vi "Solid Dilution Control-7.vi"() -> ()   [LabVIEW 2011]
uses:
  <vilib>/Instr/_visa.llb/VISA Configure Serial Port (Instr).vi
panel:
  out "(SCB) Raw":dbl
  out "Target = Soln Size?":bool=TRUE
  in  "Fill Target":dbl=450.0
  out "Hydration (g)":dbl
  in  "SIM MASS":dbl=900.0
  in  "real":bool=TRUE
  out "# of Rows Saved":i32
  in  "Tab Control":enum32{"DISPLAY", "CONFIGURE"}(tab)
  in  "Settings":T1={"ON Settings"={"Enable Dynamic Setpoint?"=TRUE, "Enable Dynamic Dispense Time?"=TRUE, "Enable Drain Rate Functions"=TRUE, "Dispense Sample Time (s)"=0.1, "Mass Average Samples"=20, "ON Timeout (sec)"=300.0, "1st Setpoint (% of Target)"=90.0, "2nd Setpoint (% of Target)"=95.0, "3rd Setpoint (% of Target)"=100.0, "Measure Dispense Delay (sec)"=10.0, "Minimum Spray Time (s)"=2.0, "Pump Reverse Time (s)"=10.0}, "OFF Settings"={"Drain Sample Time (s)"=0.1, "Drain Rate Ave Size"=100, "Drain Rate Limits (± g/sec)"=100.0, "Level Slope Range (± g/sec)"=0.05, "OFF Timeout (sec)"=300.0, "Near SP Slope Level (± g/sec)"=0.005, "Near Setpoint Threshold (%)"=99.0}, "Overshoot Settings"={"Time Limit (s)"=30.0, "Container MAX (g)"=1500.0, "Max FILL Slope (+/- g/sec)"=100.0, "% Overshot to Enable (>)"=3.0}, "FILL Timeout (s)"=300.0, "Full \nSettle Time (s)"=30.0, "Pre-Hydrate \nSpray Time (s)"=0.0, "Pre-Hydrate \nWait Time (s)"=10.0, "m Value "=1.0, "b Value"=0.0, "Enable Overshoot Adjust?"=FALSE} {"ON Settings"."Pump Reverse Time (s)" min=0.0 max=60.0; "OFF Settings"."Near SP Slope Level (± g/sec)" format="%.3g"; "OFF Settings"."Level Slope Range (± g/sec)" format="%.3g"}
  out "Values":T2 {"Drain Time (s)" format="%.2f"; "Drain Rate (g/sec)" format="%.2f"; "Spray Mass Loss (g)" format="%.2f"; "Time Elapsed (s)" format="%.2f"; "Time Target (s)" format="%.2f"; "Dynamic Setpoint (g)" format="%.2f"; "Static Setpoint (g)" format="%.2f"; "Grams to Setpoint" format="%.2f"; "Adjusted Mass (g)" format="%.2f"; "Dispense Rate (g/sec)" format="%.2f"; "Fill Mass (g)" format="%.2f"; "Fill Rate (g/sec)" format="%.2f"}
  in  "Settings Button":bool
  in  "START Dispense":bool
  in  "STOP Dispense":bool
  in  "Fill Setpoint (g)":dbl
  in  "Dispense Setpoint (%)":dbl=10.0
  out "Mass Chart":T3(graph)={"Grams (SCB)"=0.0, "Fill Target"=450.0, "Dispense Target"=0.0}
  out "Signals":T4={"Dispense"=FALSE, "Fill"=FALSE, "Spray"=FALSE, "Drain"=TRUE, "Complete"=FALSE, "Fill Error"=FALSE, "Disp. Error"=FALSE, "Fill Timeout"=FALSE, "Disp. Timeout"=FALSE, "Purge"=TRUE}
  in  "Solution Size (g)":dbl=500.0
  out "Dispense Mode":T5(ring)
  in  "Tare":bool
  out "Relay Status":T6
  in  "Save Interval (s)":dbl=1.0
  in  "Write/Read Wait (ms)":u32=100
  in  "Event Loop Wait (ms)":i32=5000
  in  "File Path Input":path
  out "SCB Error":errorcluster={"status"=TRUE, "code"=-1073807343, "source"="Property Node (arg 1) in Read SCB via ESP (SubVI).vi->Solid Dilution Control-7.vi"}
  out "SCB Output":T7
  in  "SCB COM Port":refnum<visa-resource-name>="COM5"
  in  "SCB Baud Rate":u32=9600
  out "SCB Com Error":errorcluster={"status"=TRUE, "code"=-1073807343, "source"="Property Node (arg 1) in VISA Configure Serial Port (Instr).vi->Solid Dilution Control-7.vi"}
  out "Save Error":errorcluster caption="Error Output"
  out "Weight (Grams)":dbl format="%.2f"
  out "Product Values":T8
  out "Spray Count":i32
  in  "9481 Name":tag="cDAQ3Mod1"
  out "9481 Error":errorcluster
  in  "Relay Control":T6
  out "Event Loop":i32=4
  out "Main Loop":i32=599
  out "Save Loop":i32=64
  out "DAQ/SCB Loop":i32=57
  in  "Save (Enable/Signal)":bool
  in  "STOP PROGRAM":bool
  # "SOLID DILUTION CONTROL SYSTEM"
  # "Program Last Updated 6-28-2012"
  # "SAVE\nENABLE"
  # "Blake Otting - Systems Engineering Lab - 2009"
  # "DISPENSE CONTROL"
  # "ONLY ADJUST\nBOLD VALUES!"
  # "Corrected Mass = SDC Mass * m + b"
  # "Ch0"
  # "Ch1"
  # "Ch2"
  # "Ch3"
  # "RELAY MODULE"
  # "Manual Control"
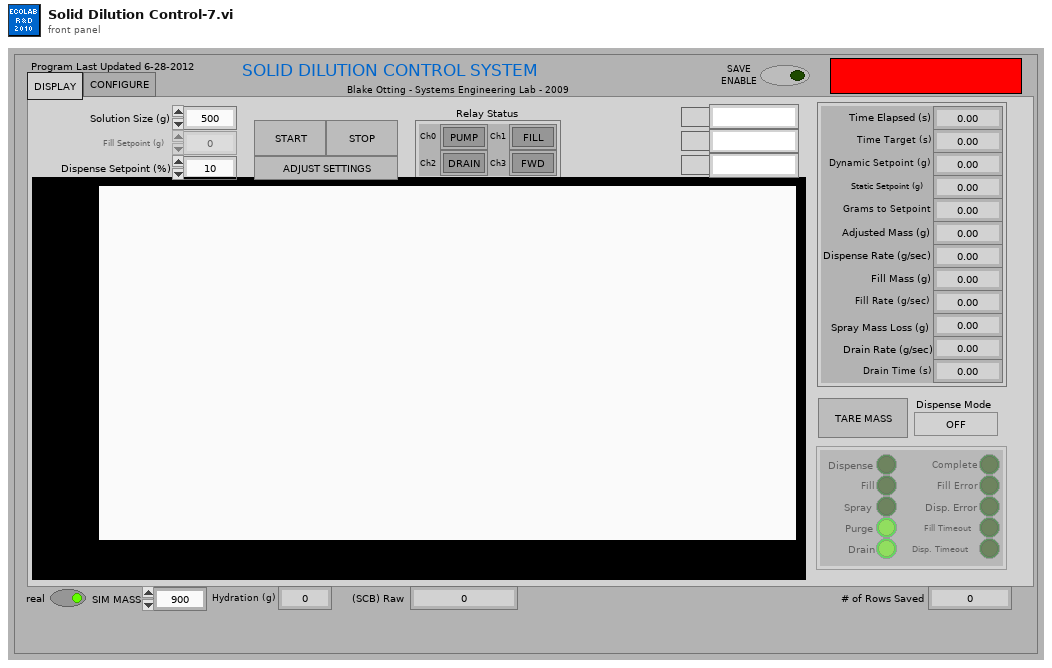
[diagram p1: front panel]
types:
  T1 = cluster{"ON Settings":cluster{"Enable Dynamic Setpoint?":bool, "Enable Dynamic Dispense Time?":bool, "Enable Drain Rate Functions":bool, "Dispense Sample Time (s)":dbl, "Mass Average Samples":i32, "ON Timeout (sec)":dbl, "1st Setpoint (% of Target)":dbl, "2nd Setpoint (% of Target)":dbl, "3rd Setpoint (% of Target)":dbl, "Measure Dispense Delay (sec)":dbl, "Minimum Spray Time (s)":dbl, "Pump Reverse Time (s)":dbl}, "OFF Settings":cluster{"Drain Sample Time (s)":dbl, "Drain Rate Ave Size":i32, "Drain Rate Limits (± g/sec)":dbl, "Level Slope Range (± g/sec)":dbl, "OFF Timeout (sec)":dbl, "Near SP Slope Level (± g/sec)":dbl, "Near Setpoint Threshold (%)":dbl}, "Overshoot Settings":cluster{"Time Limit (s)":dbl, "Container MAX (g)":dbl, "Max FILL Slope (+/- g/sec)":dbl, "% Overshot to Enable (>)":dbl}, "FILL Timeout (s)":dbl, "Full \nSettle Time (s)":dbl, "Pre-Hydrate \nSpray Time (s)":dbl, "Pre-Hydrate \nWait Time (s)":dbl, "m Value ":dbl, "b Value":dbl, "Enable Overshoot Adjust?":bool}
  T2 = cluster{"Time Elapsed (s)":dbl, "Time Target (s)":dbl, "Dynamic Setpoint (g)":dbl, "Static Setpoint (g)":dbl, "Grams to Setpoint":dbl, "Adjusted Mass (g)":dbl, "Dispense Rate (g/sec)":dbl, "Fill Mass (g)":dbl, "Fill Rate (g/sec)":dbl, "Spray Mass Loss (g)":dbl, "Drain Rate (g/sec)":dbl, "Drain Time (s)":dbl}
  T3 = cluster{"Grams (SCB)":dbl, "Fill Target":dbl, "Dispense Target":dbl}
  T4 = cluster{"Dispense":bool, "Fill":bool, "Spray":bool, "Drain":bool, "Complete":bool, "Fill Error":bool, "Disp. Error":bool, "Fill Timeout":bool, "Disp. Timeout":bool, "Purge":bool}
  T5 = enum16{"OFF", "INITIAL", "FILL", "DISPENSE", "ADJUST"}
  T6 = cluster{"PUMP ON":bool, "BASIN FILL":bool, "BASIN DRAIN":bool, "PUMP DIRECTION":bool}
  T7 = cluster{"Sequence #":string, "Weight":string, "Status":string, "CRC & EOT":string}
  T8 = cluster{"Drain Delta":dbl, "Spray Delta":dbl, "Dispense Delta":dbl}
  T9 = enum8{"Enabled", "Disabled", "Disabled and Grayed Out"}
  T10 = cluster{"Grams (SCB)":dbl, "Fill Target":dbl, "Dispense Target":dbl}[]
  T11 = cluster{"SPRAY":bool, "FILL":bool, "DRAIN":bool, "DIRECTION":bool}
  T12 = cluster{"Row Limit":i32, "Default File Name":string, "New File Daily?":bool, "Manual Save Interval?":bool}
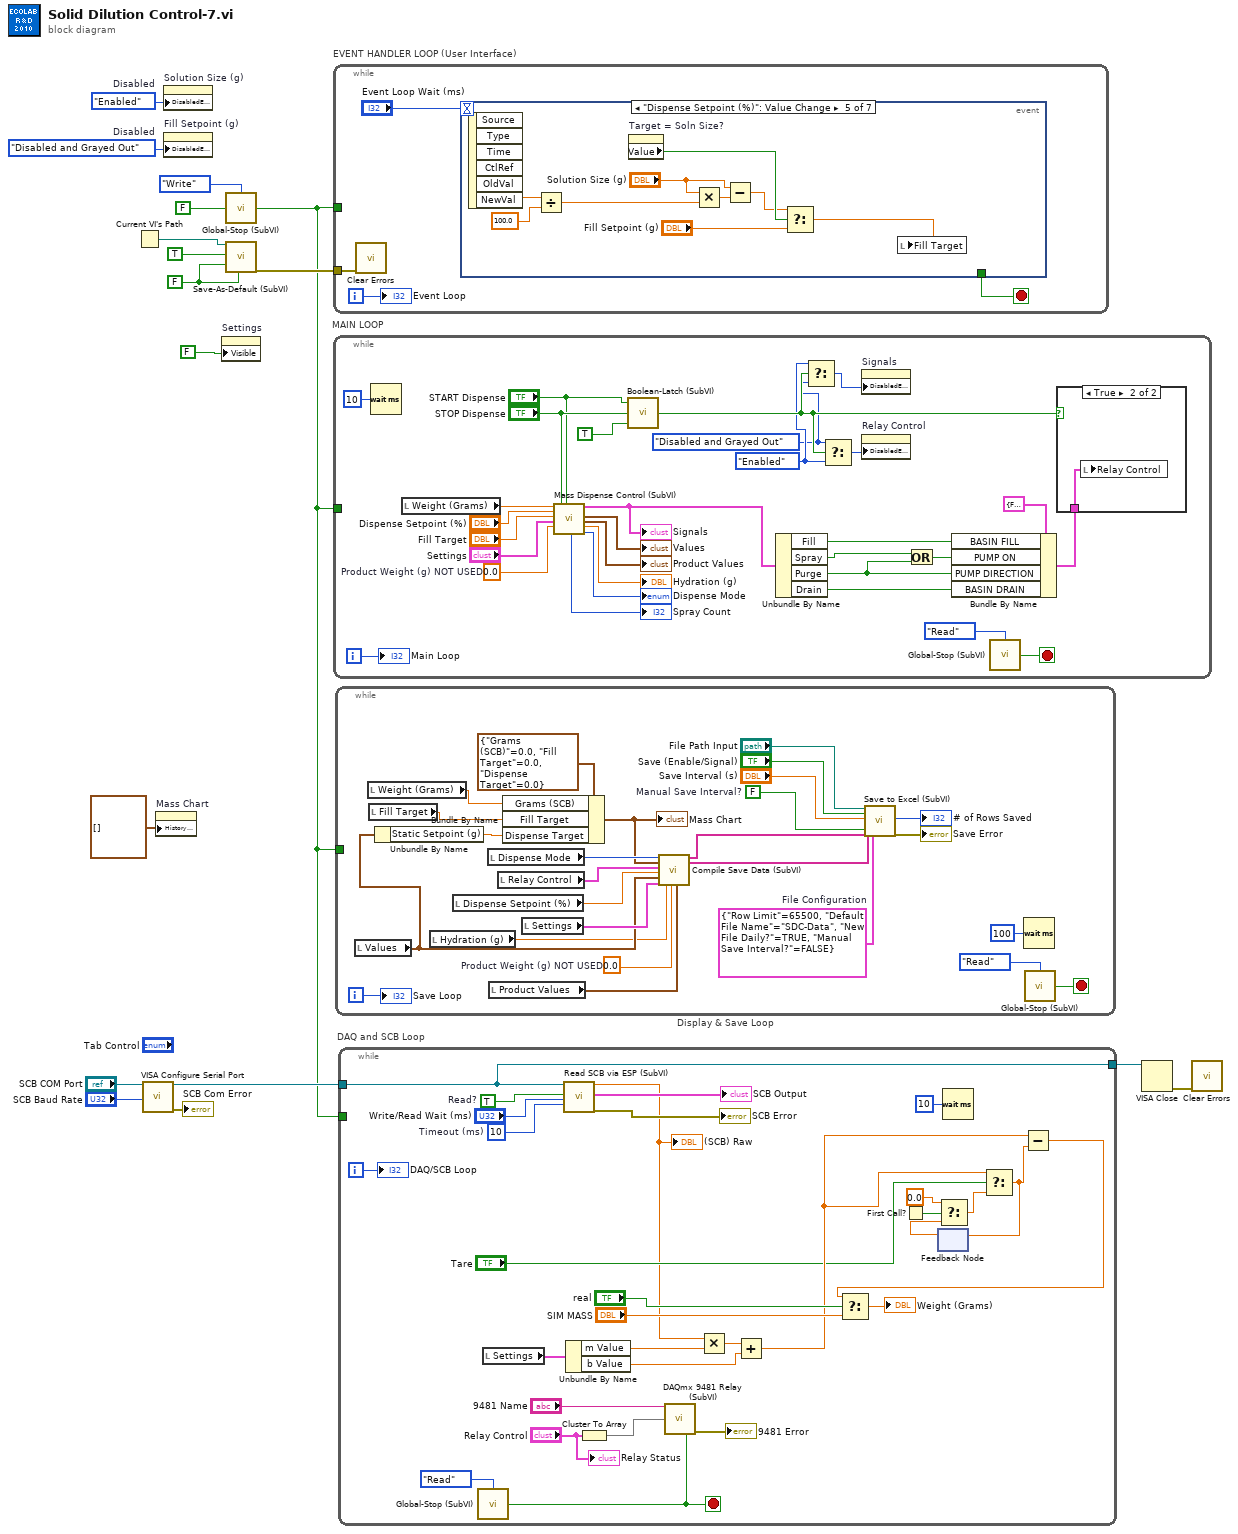
[diagram p0: block diagram]
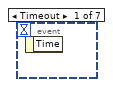
[diagram p3: hidden frame]
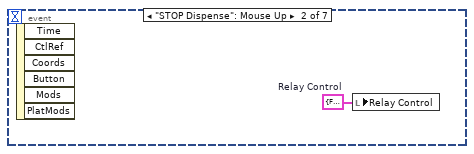
[diagram p4: hidden frame]
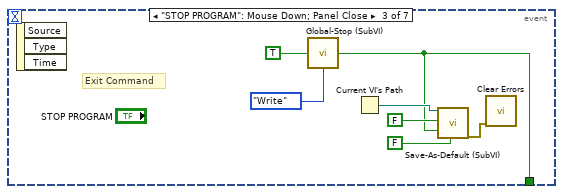
[diagram p5: hidden frame]
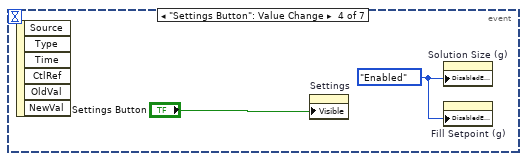
[diagram p6: hidden frame]
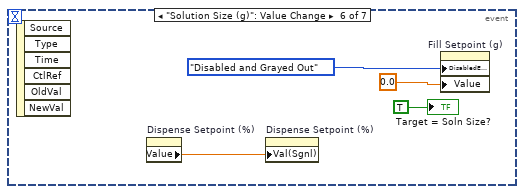
[diagram p7: hidden frame]
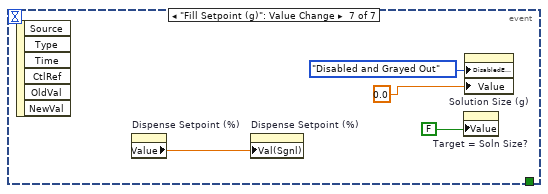
[diagram p8: hidden frame]
diagram:
  w2 = T9."Disabled and Grayed Out"  # Disabled
  w3 = T9."Enabled"  # Disabled
  w8 = FALSE ("Save Settings")
  n1 = Current VI's Path() -> (path=w10:path)
  n2 = call-poly "VISA Configure Serial Port"("VISA resource name"="SCB COM Port", "baud rate (9600)"="SCB Baud Rate") -> ("VISA resource name out"=w14:refnum<visa-resource-name>, "error out"=→"SCB Com Error":errorcluster)  [unwired: 4 in, 8 out]
  n3 = property on="Mass Chart" class="WFChart (strict)"("History Data"=T10 []) -> ()  [unwired: 2 in, 2 out]
  n4 = property on="Solution Size (g)" class="DigNum (strict)"("DisabledEnum"=w3) -> ()  [unwired: 2 in, 2 out]
  n5 = property on="Fill Setpoint (g)" class="DigNum (strict)"("DisabledEnum"=w2) -> ()  [unwired: 2 in, 2 out]
  n6 = property on="Settings" class="Clust (strict)"("Visible"=FALSE) -> ()  [unwired: 2 in, 2 out]
  n7 = call "Global-Stop (SubVI).vi"("Mode (Read)"=enum16{"Read", "Write"}."Write", "IN"=FALSE) -> ("OUT"=w4:bool)  [unwired: 2 out]
  n8 = call "Save-As-Default (SubVI).vi"("Current VI's Path"=w10, "Load Settings"=TRUE, "Save Settings"=w8, "Save and Exit"=w8) -> ("Save as Default Error"=w7:errorcluster)  [unwired: 15 in]
  n9 = while "EVENT HANDLER LOOP (User Interface)" {
    tunnel: w4 -> [_]
    tunnel: w7 -> [w19]
    i -> [w18]
    stop <- w21 stop-if-true
    n10 = call <vilib>:"Clear Errors.vi"("error in (no error)"=w19) -> ()  [unwired: 7 out]
    n11 = event shown="[4] \"Dispense Setpoint (%)\": Value Change" {
      selector: _ -> [_ _ _ _ _ _ _]
      dyn-events: _ -> [_ _ _ _ _ _ _]
      timeout: "Event Loop Wait (ms)" -> [_ _ _ _ _ _ _]
      tunnel: [_ _ w24 _ _ _ _] -> w21
      event Timeout {
        n12 = event-data() -> ()  [unwired: 2 out]
      }
      event "STOP Dispense": Mouse Up {
        w22 = T11 {"SPRAY"=FALSE, "FILL"=FALSE, "DRAIN"=FALSE, "DIRECTION"=FALSE}  # Relay Control
        n13 = event-data() -> ()  [unwired: 7 out]
        n14 = local write "Relay Control"(w22) -> ()
      }
      event "STOP PROGRAM": Mouse Down; Panel Close {
        # "Exit Command"
        n15 = event-data() -> ()  [unwired: 4 out]
        n16 = call "Global-Stop (SubVI).vi"("Mode (Read)"=enum16{"Read", "Write"}."Write", "IN"=TRUE) -> ("OUT"=w24:bool)  [unwired: 2 out]
        n17 = Current VI's Path() -> (path=w26:path)
        n18 = call "Save-As-Default (SubVI).vi"("Current VI's Path"=w26, "Load Settings"=FALSE, "Save Settings"=w24, "Save and Exit"=FALSE ("Save Settings")) -> ("Save as Default Error"=w23:errorcluster)  [unwired: 15 in]
        n19 = call <vilib>:"Clear Errors.vi"("error in (no error)"=w23) -> ()  [unwired: 7 out]
      }
      event "Settings Button": Value Change {
        w30 = T9."Enabled" ("Disabled")
        n20 = event-data() -> ()  [unwired: 7 out]
        n21 = property on="Settings" class="Clust (strict)"("Visible"="Settings Button") -> ()  [unwired: 2 in, 2 out]
        n22 = property on="Solution Size (g)" class="DigNum (strict)"("DisabledEnum"=w30) -> ()  [unwired: 2 in, 2 out]
        n23 = property on="Fill Setpoint (g)" class="DigNum (strict)"("DisabledEnum"=w30) -> ()  [unwired: 2 in, 2 out]
      }
      event "Dispense Setpoint (%)": Value Change {
        n24 = event-data() -> ("NewVal"=w39:dbl)  [unwired: 6 out]
        n25 = Divide(x=w39, y=100.0) -> (x/y=w36:dbl)
        n26 = property on="Target = Soln Size?" class="Bool (strict)"() -> ("Value"=w37:bool)  [unwired: 2 in, 2 out]
        n27 = Multiply(x="Solution Size (g)", y=w36) -> (x*y=w34:dbl)
        n28 = Subtract(x="Solution Size (g)", y=w34) -> (x-y=w33:dbl)
        n29 = Select(t=w33, s=w37, f="Fill Setpoint (g)") -> (s? t:f=w32:dbl)
        n30 = local write "Fill Target"(w32) -> ()
      }
      event "Solution Size (g)": Value Change {
        n31 = event-data() -> ()  [unwired: 7 out]
        n32 = property on="Dispense Setpoint (%)" class="DigNum (strict)"() -> ("Value"=w41:dbl)  [unwired: 2 in, 2 out]
        n33 = property on="Dispense Setpoint (%)" class="DigNum (strict)"("Val(Sgnl)"=w41) -> ()  [unwired: 2 in, 2 out]
        n34 = property on="Fill Setpoint (g)" class="DigNum (strict)"("DisabledEnum"=T9."Disabled and Grayed Out" ("Disabled"), "Value"=0.0 ("Fill Setpoint (g)")) -> ()  [unwired: 2 in, 2 out]
        "Target = Soln Size?" <- TRUE
      }
      event "Fill Setpoint (g)": Value Change {
        n35 = event-data() -> ()  [unwired: 7 out]
        n36 = property on="Dispense Setpoint (%)" class="DigNum (strict)"() -> ("Value"=w45:dbl)  [unwired: 2 in, 2 out]
        n37 = property on="Dispense Setpoint (%)" class="DigNum (strict)"("Val(Sgnl)"=w45) -> ()  [unwired: 2 in, 2 out]
        n38 = property on="Target = Soln Size?" class="Bool (strict)"("Value"=FALSE) -> ()  [unwired: 2 in, 2 out]
        n39 = property on="Solution Size (g)" class="DigNum (strict)"("DisabledEnum"=T9."Disabled and Grayed Out" ("Disabled"), "Value"=0.0 ("Fill Setpoint (g)")) -> ()  [unwired: 2 in, 2 out]
      }
    }
    "Event Loop" <- w18
  }
  n40 = while "MAIN LOOP" {
    tunnel: w4 -> [_]
    i -> [w75]
    stop <- w76 stop-if-true
    w56 = T9."Enabled"
    w55 = T9."Disabled and Grayed Out"
    w62 = 0.0  # Product Weight (g) NOT USED
    n41 = Wait (ms)(milliseconds to wait=u32 10) -> ()  [unwired: 1 out]
    n42 = local read "Weight (Grams)"() -> (w69:dbl)
    n43 = call "Mass Dispense Control (SubVI).vi"("Weight (Grams)"=w69, "Dispense Setpoint (%)"="Dispense Setpoint (%)", "Fill Setpoint (g)"="Fill Target", "Settings"="Settings", "Product Weight (g)"=w62, "STOP Dispense"="STOP Dispense", "START Dispense"="START Dispense") -> ("Spray Count"=→"Spray Count":i32, "Signals"=w61:T4, "Values"=→"Values":T2, "Product Values"=→"Product Values":T8, "Hydration (g)"=→"Hydration (g)":dbl, "Dispense Mode"=→"Dispense Mode":T5)  [unwired: 1 in, 6 out]
    "Signals" <- w61
    n44 = call "Boolean-Latch (SubVI).vi"("Reset on First Call (T)"=TRUE, "Reset"="STOP Dispense", "Trigger (Input)"="START Dispense") -> ("Latched? (Output)"=w57:bool)
    n45 = Unbundle By Name(w61) -> ("Fill"=w60:bool, "Spray"=w53:bool, "Purge"=w51:bool, "Drain"=w49:bool)
    n46 = Select(t=w56, s=w57, f=w55) -> (s? t:f=w54:T9)
    n47 = Select(t=w55, s=w57, f=w56) -> (s? t:f=w58:T9)
    n48 = property on="Signals" class="Clust (strict)"("DisabledEnum"=w54) -> ()  [unwired: 2 in, 2 out]
    n49 = property on="Relay Control" class="Clust (strict)"("DisabledEnum"=w58) -> ()  [unwired: 2 in, 2 out]
    n50 = Or(x=w53, y=w51) -> (x .or. y?=w52:bool)
    n51 = Bundle By Name(cluster=T6 {"PUMP ON"=FALSE, "BASIN FILL"=FALSE, "BASIN DRAIN"=FALSE, "PUMP DIRECTION"=FALSE}, "BASIN FILL"=w60, "PUMP ON"=w52, "PUMP DIRECTION"=w51, "BASIN DRAIN"=w49) -> (w59:T6)
    n52 = call "Global-Stop (SubVI).vi"("Mode (Read)"=enum16{"Read", "Write"}."Read") -> ("OUT"=w76:bool)  [unwired: 1 in, 2 out]
    n53 = case shown="True" w57 {
      tunnel: w59 -> [_ w79]
      frame False {
      }
      frame True {
        n54 = local write "Relay Control"(w79) -> ()
      }
    }
    "Main Loop" <- w75
  }
  n55 = while "Display & Save Loop" {
    tunnel: w4 -> [_]
    i -> [w96]
    stop <- w103 stop-if-true
    w81 = 0.0  # Product Weight (g) NOT USED
    w84 = T12 {"Row Limit"=65500, "Default File Name"="SDC-Data", "New File Daily?"=TRUE, "Manual Save Interval?"=FALSE}  # File Configuration
    w98 = FALSE  # Manual Save Interval?
    n56 = local read "Values"() -> (w88:T2)
    n57 = local read "Weight (Grams)"() -> (w90:dbl)
    n58 = local read "Fill Target"() -> (w82:dbl)
    n59 = Unbundle By Name(w88) -> ("Static Setpoint (g)"=w94:dbl)
    n60 = local read "Hydration (g)"() -> (w85:dbl)
    n61 = local read "Dispense Setpoint (%)"() -> (w92:dbl)
    n62 = local read "Dispense Mode"() -> (w89:T5)
    n63 = local read "Product Values"() -> (w86:T8)
    n64 = local read "Relay Control"() -> (w80:T6)
    n65 = Bundle By Name(cluster=T3 {"Grams (SCB)"=0.0, "Fill Target"=0.0, "Dispense Target"=0.0} ("Conductivity"), "Grams (SCB)"=w90, "Fill Target"=w82, "Dispense Target"=w94) -> (w87:T3)
    "Mass Chart" <- w87
    n66 = local read "Settings"() -> (w91:T1)
    n67 = call "Compile Save Data (SubVI).vi"("Dispense Mode"=w89, "Mass Chart"=w87, "Relay Control"=w80, "Dispense Setpoint (%)"=w92, "Values"=w88, "Settings"=w91, "Hydration (g)"=w85, "Product Mass (g)"=w81, "Product Values"=w86) -> ("Data Array Output"=w83:string[], "Column Header Text Array"=w93:string[])  [unwired: 9 out]
    n68 = call "Save to Excel (SubVI).vi"("File Path Input"="File Path Input", "Save (Enable/Signal)"="Save (Enable/Signal)", "Save Interval (s)"="Save Interval (s)", "Column Header Array"=w93, "Data Array (Row)"=w83, "File Configuration"=w84, "Change Save Location?"=w98) -> ("# of Rows Saved"=→"# of Rows Saved":i32, "Error Output"=→"Save Error":errorcluster)  [unwired: 8 in, 3 out]
    n69 = Wait (ms)(milliseconds to wait=u32 100) -> ()  [unwired: 1 out]
    n70 = call "Global-Stop (SubVI).vi"("Mode (Read)"=enum16{"Read", "Write"}."Read") -> ("OUT"=w103:bool)  [unwired: 1 in, 2 out]
    "Save Loop" <- w96
  }
  n71 = while "DAQ and SCB Loop" {
    tunnel: w14 -> [w128]
    tunnel: [w128] -> w11
    tunnel: w4 -> [_]
    i -> [w127]
    stop <- w120 stop-if-true
    w135 = TRUE  # Read?
    w133 = u32 10  # Timeout (ms)
    n72 = call "Global-Stop (SubVI).vi"("Mode (Read)"=enum16{"Read", "Write"}."Read") -> ("OUT"=w120:bool)  [unwired: 1 in, 2 out]
    n73 = local read "Settings"() -> (w119:T1)
    n74 = call "Read SCB via ESP (SubVI).vi"("COM Port Input"=w128, "Manual Write Command"=w135, "Write/Read Wait (ms)"="Write/Read Wait (ms)", "Timeout (ms)"=w133) -> ("Weight (Grams)"=w108:dbl, "SCB Output"=→"SCB Output":T7, "Error Output"=→"SCB Error":errorcluster)  [unwired: 1 in, 12 out]
    "(SCB) Raw" <- w108
    n75 = Unbundle By Name(w119) -> ("m Value"=w118:dbl, "b Value"=w116:dbl)
    n76 = Cluster To Array(cluster="Relay Control") -> (array=w121:bool[])
    n77 = call "DAQmx 9481 Relay (SubVI).vi"("9481 Name"="9481 Name", "Relay Control"=w121, "Stop Program"=w120) -> ("Relay Error"=→"9481 Error":errorcluster)  [unwired: 12 in]
    n78 = Multiply(x=w108, y=w118) -> (x*y=w117:dbl)
    n79 = Add(x=w117, y=w116) -> (x+y=w115:dbl)
    n80 = First Call?() -> (First Call?: T/F=w113:bool)
    n81 = feedback #1() -> (w110:dbl)  [unwired: 1 in]
    n82 = Select(t=0.0, s=w113, f=w110) -> (s? t:f=w112:dbl)
    n83 = Wait (ms)(milliseconds to wait=u32 10) -> ()  [unwired: 1 out]
    n84 = Select(t=w115, s="Tare", f=w112) -> (s? t:f=w111:dbl)
    n85 = feedback-in #1(w111) -> ()
    n86 = Subtract(x=w115, y=w111) -> (x-y=w107:dbl)
    n87 = Select(t=w107, s="real", f="SIM MASS") -> (s? t:f=→"Weight (Grams)":dbl)
    "DAQ/SCB Loop" <- w127
    "Relay Status" <- "Relay Control"
  }
  n88 = VISA Close(VISA resource name=w11) -> (error out=w1:errorcluster)  [unwired: 1 in]
  n89 = call <vilib>:"Clear Errors.vi"("error in (no error)"=w1) -> ()  [unwired: 6 in, 1 out]
